vi "Read Orig Anal Setup.vi"(3 "Use Analogue channel to software sync with LDA":bool, 5 "Setup string":string) -> (1 "Ch & spans choices":T2[](array[typedef]) {"Fs" format="%#_pHz"; "syncDelay" format="%#_gms"; "Ch" min=0 step=1}, 2 "Number of Analogue instruments":i32=1)   [LabVIEW 2022 SP3]
uses:
  Controls/Inst_type.ctl
  Controls/Post_Process.ctl
  Globals/Meas_global.vi
  Controls/portOrDev.ctl
  Controls/calType.ctl
  Controls/channelState.ctl
  Controls/Meas input Cluster.ctl
panel:
  in  "Inst type":T1=enum."Propeller anemometer"
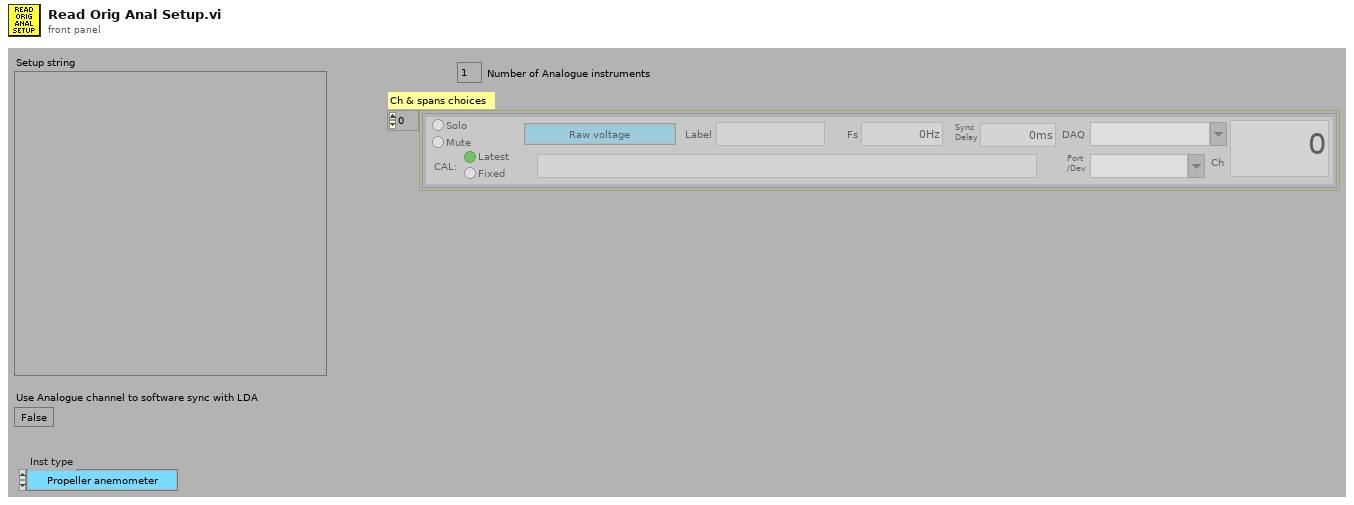
[diagram p1: front panel]
types:
  T1 = typedef "Inst_type.ctl" = enum16{"Raw voltage", "Raw with zero offsetting", "Propeller anemometer", "Pressure Transducer", "Pitot-static tube", "Hot wire", "Cross wire 1", "Cross wire 2", "Generic Linear", "Generic Polynomial", "Generic BackPoly", "Fast FID", "Thermocouple", "Cold wire", "Pulsed Wire", "LDA Vel", "LDA Tran time", "LDA Arr time", "Microphone"}
  T2 = typedef "Meas input Cluster.ctl" = cluster{"Type":T1, "Label":string, "DAQ":string, "Port":T3, "Ch":i32, "Cal":path, "calType":T4, "Fs":dbl, "syncDelay":dbl, "chState":T5}
  T3 = typedef "portOrDev.ctl" = string
  T4 = typedef "calType.ctl" = enum32{"Latest", "Fixed"}
  T5 = typedef "channelState.ctl" = enum32{"No Selection", "Solo", "Mute"}
  T6 = typedef "Post_Process.ctl" = enum16{"Take New Data", "Post Process Raw Data File"}
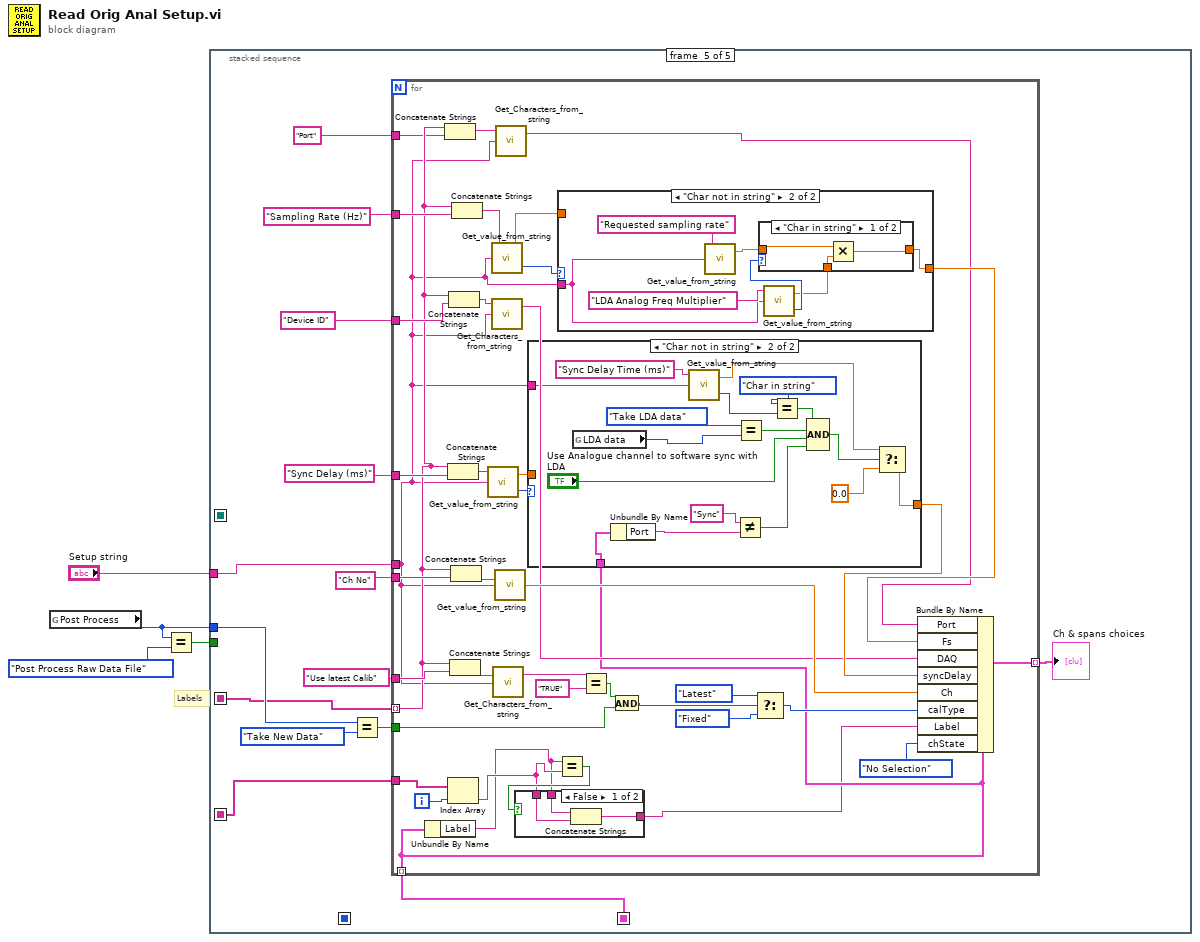
[diagram p0: block diagram]
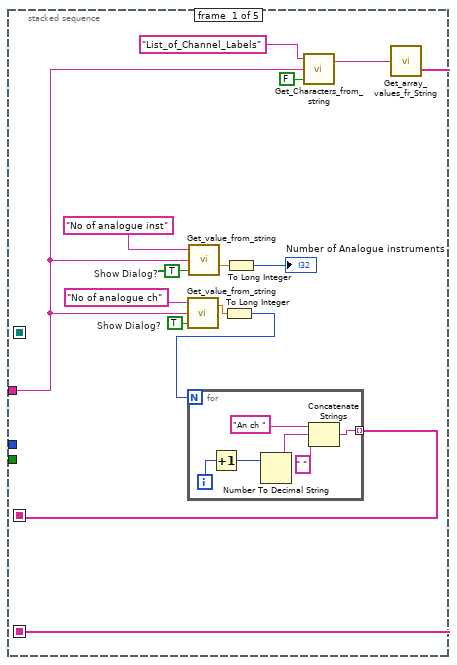
[diagram p2: hidden frame]
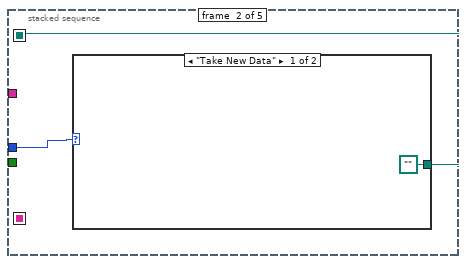
[diagram p3: hidden frame]
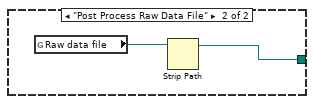
[diagram p4: hidden frame]
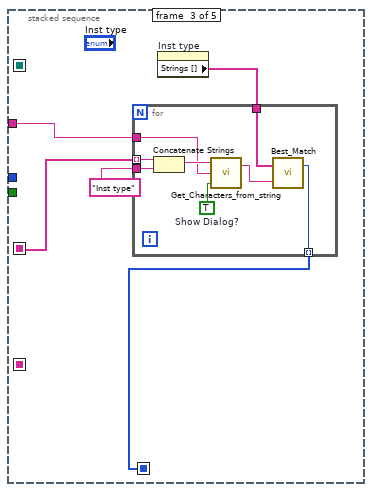
[diagram p5: hidden frame]
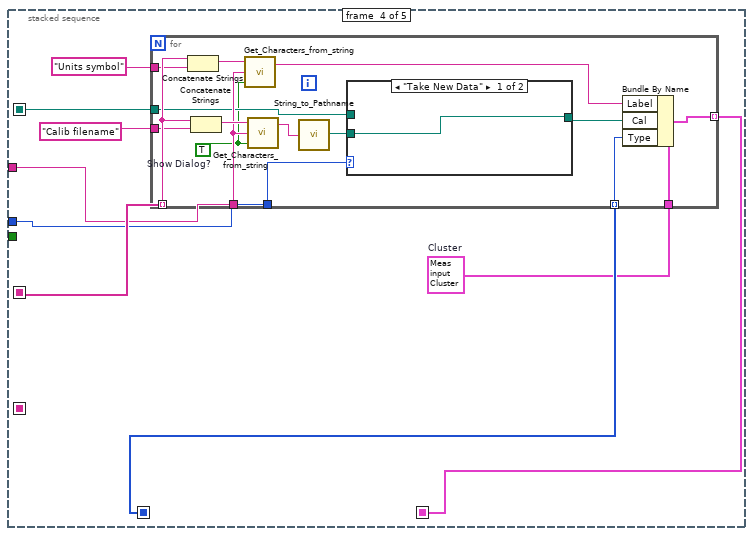
[diagram p6: hidden frame]
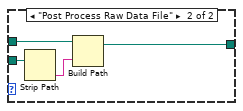
[diagram p7: hidden frame]
diagram:
  # "Labels"
  n1 = global read "Meas_global.vi" "Post Process"() -> (w2:T6)
  n2 = Equal?(x=w2, y=Post_Process."Post Process Raw Data File" ("Post Process")) -> (x = y?=w4:bool)
  n3 = stacked-sequence {
    seq-local: [w16 _ _ _ _] -> [_ _ w34 w51 w79]
    seq-local: [_ _ w31 _ _] -> [_ _ _ w48 _]
    seq-local: [_ _ _ w47 _] -> [_ _ _ _ w86]
    seq-local: [_ w26 _ _ _] -> [_ _ _ w46 _]
    seq-local: [w6 _ _ _ _] -> [_ _ _ _ w74]
    tunnel: w4 -> [_ _ _ _ _]
    tunnel: w2 -> [_ w25 _ w45 w80]
    tunnel: "Setup string" -> [w5 _ w30 w44 w73]
    frame #0 {
      w10 = TRUE  # Show Dialog?
      w11 = TRUE  # Show Dialog?
      n4 = call "Get_value_from_string.vi"("Show Dialog?"=w11, "Input string"=w5, "Variable name"="No of analogue ch") -> ("Value"=w17:dbl)  [unwired: 1 out]
      n5 = call "Get_value_from_string.vi"("Show Dialog?"=w10, "Input string"=w5, "Variable name"="No of analogue inst") -> ("Value"=w14:dbl)  [unwired: 1 out]
      n6 = To Long Integer(number=w17) -> (32bit integer=w12:i32)
      n7 = for {
        N: w12 -> [_]
        tunnel: [w20] -> w16 mode=indexing
        i -> [w22]
        n8 = Increment(x=w22) -> (x+1=w21:i32)
        n9 = Number To Decimal String(number=w21) -> (decimal integer string=w24:string)  [unwired: 1 out]
        n10 = Concatenate Strings("An ch ", w24, " ") -> (w20:string)
      }
      n11 = To Long Integer(number=w14) -> (32bit integer=→"Number of Analogue instruments":i32)
      n12 = call "Get_Characters_from_string.vi"("Show Dialog?"=FALSE, "Input string"=w5, "Variable name"="List_of_Channel_Labels") -> ("Value"=w7:string)  [unwired: 1 out]
      n13 = call "Get_array_values_fr_String.vi"("String Value"=w7) -> ("String array"=w6:string[])  [unwired: 1 out]
    }
    frame #1 {
      n14 = case shown="\"Take New Data\"" w25 {
        tunnel: [path "" ("stripped path") w28] -> w26
        frame "Take New Data" {
        }
        frame "Post Process Raw Data File" {
          n15 = global read "Meas_global.vi" "Raw data file"() -> (w29:path)
          n16 = Strip Path(path=w29) -> (stripped path=w28:path)  [unwired: 1 out]
        }
      }
    }
    frame #2 {
      n17 = property on="Inst type" class="Enum (strict)"() -> ("Strings []"=w32:string[])  [unwired: 2 in, 2 out]
      n18 = for {
        tunnel: w30 -> [w41]
        tunnel: w32 -> [w37]
        tunnel: w34 -> [w40] mode=indexing
        tunnel: "Inst type" -> [w39]
        tunnel: [w35] -> w31 mode=indexing
        w38 = TRUE  # Show Dialog?
        n19 = Concatenate Strings(w40, w39) -> (w42:string)
        n20 = call "Get_Characters_from_string.vi"("Show Dialog?"=w38, "Input string"=w41, "Variable name"=w42) -> ("Value"=w36:string)  [unwired: 1 out]
        n21 = call "Best_Match.vi"("Input String"=w36, "String Options"=w37) -> ("index of element"=w35:i32)  [unwired: 1 out]
      }
    }
    frame #3 {
      w43 = T2 {"Type"=enum."Raw voltage", "Label"="", "DAQ"="", "Port"="", "Ch"=0, "Cal"=path "", "calType"=enum."Latest", "Fs"=0.0, "syncDelay"=0.0, "chState"=enum."No Selection"}  # Cluster
      n22 = for {
        tunnel: w51 -> [w65] mode=indexing
        tunnel: "Calib filename" -> [w64]
        tunnel: "Units symbol" -> [w63]
        tunnel: w43 -> [w62]
        tunnel: w48 -> [w60] mode=indexing
        tunnel: [w59] -> w47 mode=indexing
        tunnel: w44 -> [w58]
        tunnel: w45 -> [w57]
        tunnel: w46 -> [w56]
        w54 = TRUE  # Show Dialog?
        n23 = Concatenate Strings(w65, w63) -> (w67:string)
        n24 = Concatenate Strings(w65, w64) -> (w66:string)
        n25 = call "Get_Characters_from_string.vi"("Show Dialog?"=w54, "Input string"=w58, "Variable name"=w67) -> ("Value"=w61:string)  [unwired: 1 out]
        n26 = call "Get_Characters_from_string.vi"("Show Dialog?"=w54, "Input string"=w58, "Variable name"=w66) -> ("Value"=w53:string)  [unwired: 1 out]
        n27 = call "String_to_Pathname.vi"("Input String"=w53) -> ("path"=w52:path)
        n28 = case shown="\"Take New Data\"" w57 {
          tunnel: w52 -> [w68 w72]
          tunnel: w56 -> [_ w69]
          tunnel: [w68 w70] -> w55
          frame "Take New Data" {
          }
          frame "Post Process Raw Data File" {
            n29 = Strip Path(path=w72) -> (name=w71:string)  [unwired: 1 out]
            n30 = Build Path(base path=w69, name or relative path=w71) -> (appended path=w70:path)
          }
        }
        n31 = Bundle By Name(cluster=w62, "Label"=w61, "Cal"=w55, "Type"=w60) -> (w59:T2)
      }
    }
    frame #4 {
      n32 = Equal?(x=w80, y=Post_Process."Take New Data" ("Post Process")) -> (x = y?=w78:bool)
      n33 = for {
        tunnel: "Sync Delay (ms)" -> [w126]
        tunnel: w86 -> [w92] mode=indexing
        tunnel: [w121] -> w85 mode=indexing
        tunnel: w73 -> [w99]
        tunnel: "Ch No" -> [w123]
        tunnel: "Use latest Calib" -> [w119]
        tunnel: w79 -> [w103] mode=indexing
        tunnel: w78 -> [w115]
        tunnel: "Device ID" -> [w109]
        tunnel: "Sampling Rate (Hz)" -> [w107]
        tunnel: "Port" -> [w102]
        tunnel: w74 -> [w98]
        i -> [w97]
        n34 = Unbundle By Name(w92) -> ("Label"=w89:string)
        n35 = Concatenate Strings(w103, w102) -> (w101:string)
        n36 = Concatenate Strings(w103, w126) -> (w125:string)
        n37 = Index Array(array=w98, index=w97) -> (element=w90:string)
        n38 = Concatenate Strings(w103, w109) -> (w110:string)
        n39 = Concatenate Strings(w103, w119) -> (w120:string)
        n40 = Concatenate Strings(w103, w123) -> (w124:string)
        n41 = Concatenate Strings(w103, w107) -> (w108:string)
        n42 = call "Get_value_from_string.vi"("Input string"=w99, "Variable name"=w125) -> ("Status"=w114:enum16{"Char in string", "Char not in string"}, "Value"=w112:dbl)  [unwired: 1 in]
        n43 = call "Get_value_from_string.vi"("Input string"=w99, "Variable name"=w108) -> ("Status"=w106:enum16{"Char in string", "Char not in string"}, "Value"=w104:dbl)  [unwired: 1 in]
        n44 = call "Get_Characters_from_string.vi"("Input string"=w99, "Variable name"=w110) -> ("Value"=w111:string)  [unwired: 1 in, 1 out]
        n45 = call "Get_Characters_from_string.vi"("Input string"=w99, "Variable name"=w120) -> ("Value"=w118:string)  [unwired: 1 in, 1 out]
        n46 = call "Get_value_from_string.vi"("Input string"=w99, "Variable name"=w124) -> ("Value"=w122:dbl)  [unwired: 1 in, 1 out]
        n47 = call "Get_Characters_from_string.vi"("Input string"=w99, "Variable name"=w101) -> ("Value"=w100:string)  [unwired: 1 in, 1 out]
        n48 = case shown="\"Char not in string\"" w114 {
          tunnel: [w143 w156] -> w113
          tunnel: w112 -> [w143 _]
          tunnel: w92 -> [_ w155]
          tunnel: w99 -> [_ w151]
          frame "Char in string" {
          }
          frame "Char not in string" {
            n49 = global read "Meas_global.vi" "LDA data"() -> (w145:enum16{"No LDA data", "Take LDA data"})
            n50 = Unbundle By Name(w155) -> ("Port"=w154:T3)
            n51 = call "Get_value_from_string.vi"("Input string"=w151, "Variable name"="Sync Delay Time (ms)" ("Label for characters")) -> ("Status"=w147:enum16{"Char in string", "Char not in string"}, "Value"=w149:dbl)  [unwired: 1 in]
            n52 = Not Equal?(x="Sync", y=w154) -> (x != y?=w152:bool)
            n53 = Equal?(x=enum16{"No LDA data", "Take LDA data"}."Take LDA data", y=w145) -> (x = y?=w159:bool)
            n54 = Equal?(x=enum16{"Char in string", "Char not in string"}."Char in string" ("Status"), y=w147) -> (x = y?=w146:bool)
            n55 = Compound Arithmetic op=AND(w146, w159, "Use Analogue channel to software sync with LDA", w152) -> (w158:bool)
            n56 = Select(t=w149, s=w158, f=0.0) -> (s? t:f=w156:dbl)
          }
        }
        n57 = Equal?(x=w89, y=w90) -> (x = y?=w91:bool)
        n58 = case shown="False" w91 {
          tunnel: [w127 w130] -> w88
          tunnel: w90 -> [w128 w130]
          tunnel: w89 -> [w129 _]
          frame False {
            n59 = Concatenate Strings(w129, w128) -> (w127:string)
          }
          frame True {
          }
        }
        n60 = case shown="\"Char not in string\"" w106 {
          tunnel: [w131 w134] -> w105
          tunnel: w104 -> [w131 _]
          tunnel: w99 -> [_ w136]
          frame "Char in string" {
          }
          frame "Char not in string" {
            n61 = call "Get_value_from_string.vi"("Input string"=w136, "Variable name"="Requested sampling rate") -> ("Value"=w133:dbl)  [unwired: 1 in, 1 out]
            n62 = call "Get_value_from_string.vi"("Input string"=w136, "Variable name"="LDA Analog Freq Multiplier") -> ("Status"=w135:enum16{"Char in string", "Char not in string"}, "Value"=w132:dbl)  [unwired: 1 in]
            n63 = case shown="\"Char in string\"" w135 {
              tunnel: [w139 w142] -> w134
              tunnel: w133 -> [w141 w142]
              tunnel: w132 -> [w140 _]
              frame "Char in string" {
                n64 = Multiply(x=w141, y=w140) -> (x*y=w139:dbl)
              }
              frame "Char not in string" {
              }
            }
          }
        }
        n65 = Equal?(x=w118, y="TRUE") -> (x = y?=w116:bool)
        n66 = And(x=w116, y=w115) -> (x .and. y?=w94:bool)
        n67 = Select(t=calType."Latest" ("calType"), s=w94, f=calType."Fixed" ("calType")) -> (s? t:f=w93:T4)
        n68 = Bundle By Name(cluster=w92, "Port"=w100, "Fs"=w105, "DAQ"=w111, "syncDelay"=w113, "Ch"=w122, "calType"=w93, "Label"=w88, "chState"=channelState."No Selection") -> (w121:T2)
      }
      "Ch & spans choices" <- w85
    }
  }
